vi "FlatToRichrfcontrol_SetGPSUTCStartTimeRequest.vi"(5 "OutputClusterType":T1, 11 "InputCluster":T2) -> (3 "OutputCluster":T1)   [LabVIEW 2024, in "FlexSDR_gRPC_client.lvlib"]
uses:
  rfcontrol_SetGPSUTCStartTimeRequest_Flat.ctl
  rfcontrol_SetGPSUTCStartTimeRequest.ctl
  FlexSDR_gRPC_client.lvlib
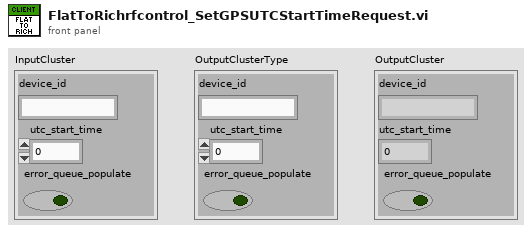
[diagram p1: front panel]
types:
  T1 = typedef "FlexSDR_gRPC_client.lvlib/rfcontrol_SetGPSUTCStartTimeRequest.ctl" = cluster{"device_id":string, "utc_start_time":dbl, "error_queue_populate":bool}
  T2 = typedef "FlexSDR_gRPC_client.lvlib/rfcontrol_SetGPSUTCStartTimeRequest_Flat.ctl" = cluster{"device_id":string, "utc_start_time":dbl, "error_queue_populate":bool}
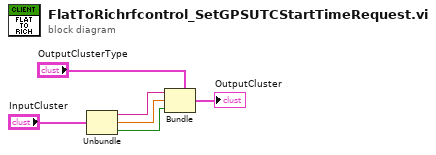
[diagram p0: block diagram]
diagram:
  n1 = Unbundle "Unbundle"("InputCluster") -> ("device_id"=w3:string, "utc_start_time"=w2:dbl, "error_queue_populate"=w1:bool)
  n2 = Bundle "Bundle"(cluster="OutputClusterType", "device_id"=w3, "utc_start_time"=w2, "error_queue_populate"=w1) -> (→"OutputCluster":T1)
